vi "read_volume_set.vi"(8 "error in":errorcluster, 11 "binary folder":path) -> (0 "error out":errorcluster, 2 "matched set":set{cluster{"CLZ id":i32, "CV id":i32}}(c389))   [LabVIEW 2024, in "CLZ_to_ComicVine.lvlib"]
uses:
  CLZ_to_ComicVine.lvlib
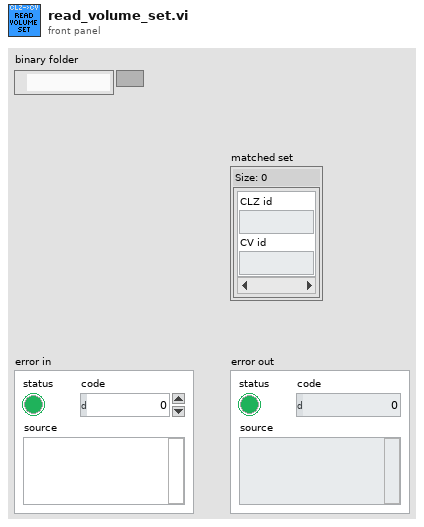
[diagram p1: front panel]
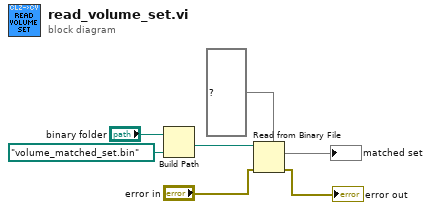
[diagram p0: block diagram]
diagram:
  n1 = Build Path(base path="binary folder", name or relative path=path "volume_matched_set.bin") -> (appended path=w5:path)
  n2 = Read from Binary File(5:set{cluster{"CLZ id":i32, "CV id":i32}} {} ("matched set"), 8:"error in", 11:w5) -> (0:→"error out":errorcluster, 2:→"matched set":set{cluster{"CLZ id":i32, "CV id":i32}})  [unwired: 3 in, 2 out]
